vi "Get BC.vi"(8 "error in (no error)":errorcluster, 10 "Domain":refnum<class "NI_Domain.lvclass">, 11 "BC_Steady_2D_Numeric in":refnum<class "NI_BC_Steady_2D_Numeric.lvclass">) -> (0 "error out":errorcluster, 2 "BC":variant, 3 "BC_Steady_2D_Numeric out":refnum<class "NI_BC_Steady_2D_Numeric.lvclass">)   [LabVIEW 2020, in "NI_PDE.lvlib" / "NI_BC_Steady_2D_Numeric.lvclass"]
uses:
  <vilib>/gmath/pde.llb/BCClass/BC_Steady_2D_Numeric/NI_BC_Steady_2D_Numeric.lvclass
  <vilib>/gmath/pde.llb/DomainClass/NI_Domain.lvclass
  <vilib>/gmath/pde.llb/BCClass/BC_Steady_2D_Numeric/BC Data.ctl
  <vilib>/gmath/pde.llb/Common/PDE_BC Type.ctl
  <vilib>/gmath/pde.llb/Common/PDE_BC Position 2D.ctl
  <vilib>/gmath/pde.llb/BCClass/BC_Steady_2D_Numeric/NI_BC_Steady_2D_Numeric.lvclass/NI_BC_Steady_2D_Numeric.ctl
  <vilib>/gmath/NI_PDE.lvlib
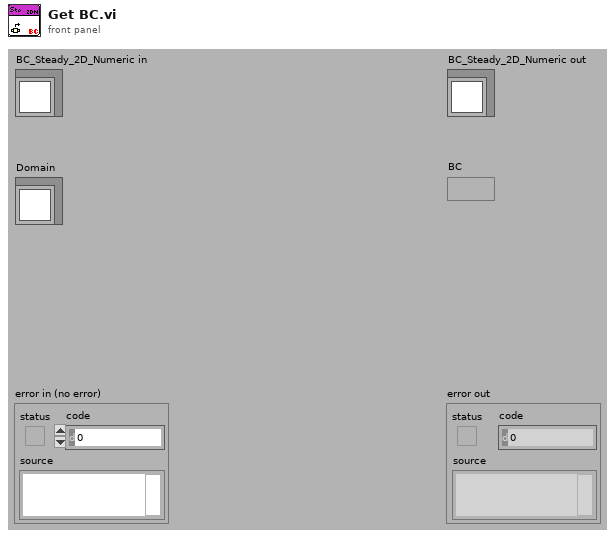
[diagram p1: front panel]
types:
  T1 = typedef "NI_PDE.lvlib/NI_BC_Steady_2D_Numeric.lvclass/BC Data.ctl" = cluster{"type":T2, "position":T3, "G":dbl[]}
  T2 = typedef "NI_PDE.lvlib/PDE_BC Type.ctl" = i32
  T3 = typedef "NI_PDE.lvlib/PDE_BC Position 2D.ctl" = i32
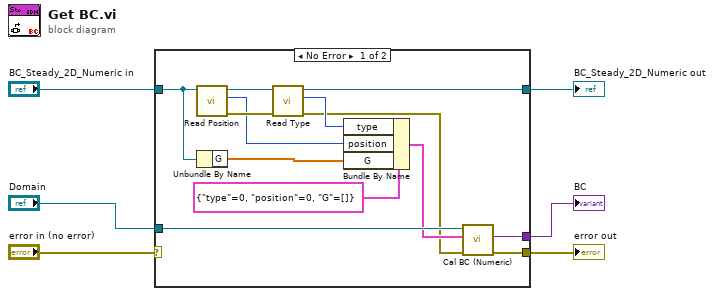
[diagram p0: block diagram]
diagram:
  n1 = case shown="No Error" "error in (no error)" {
    selector: "error in (no error)" -> [_ w21]
    tunnel: "BC_Steady_2D_Numeric in" -> [w16 w20]
    tunnel: [w18 _] -> w3
    tunnel: [w14 w20] -> w6
    tunnel: [w17 w21] -> w4
    tunnel: "Domain" -> [w19 _]
    frame No Error {
      n2 = call-dynamic "Read Position.vi"("BC_Steady_2D.lvclass in"=w16) -> ("error out"=w13:errorcluster, "BC position 2D"=w10:T3, "BC_Steady_2D.lvclass out"=w15:refnum<class "NI_BC_Steady_2D_Numeric.lvclass">)  [unwired: 1 in, 7 out]
      n3 = Unbundle By Name(w16) -> ("G"=w9:dbl[])
      n4 = call-dynamic "Read Type.vi"("error in (no error)"=w13, "BC.lvclass in"=w15) -> ("error out"=w7:errorcluster, "BC type"=w11:T2, "BC.lvclass out"=w14:refnum<class "NI_BC_Steady_2D_Numeric.lvclass">)  [unwired: 7 out]
      n5 = Bundle By Name(cluster=T1 {"type"=0, "position"=0, "G"=[]} ("BC data"), "type"=w11, "position"=w10, "G"=w9) -> (w8:T1)
      n6 = call-dynamic "Cal BC (Numeric).vi"("error in (no error)"=w7, "BC in"=w8, "Domain in"=w19) -> ("error out"=w17:errorcluster, "BC out"=w18:variant)  [unwired: 7 out]
    }
    frame Error {
    }
  }
  "BC" <- w3
  "error out" <- w4
  "BC_Steady_2D_Numeric out" <- w6
